vi "IDS-3060-control.vi"() -> ()   [LabVIEW 2014]
uses:
  <vilib>/Analysis/NI_AALBase.lvlib
panel:
  in  "Save image":bool
  in  "File name":string="img"
  in  "Folder Path":path=path "D:/Images/asd"
  in  "zoom":dbl(slide)=0.9914131207450079 scale=0.1..5.0
  in  "height":dbl(slide)=1272.7748691099475 scale=0.0..1300.0
  in  "width":dbl(slide)=2000.0 scale=0.0..2000.0
  out "white leve":u8=255
  out "black levell":u8
  in  "Slide":cluster{u8, u8}(slide)={0, 255} scale=0.0..255.0
  out "SizeOut":T1
  in  "stop":bool
  out "error out":errorcluster
  in  "Exposure[ms]":dbl=20.0 format="%#_13g"
  out "Hist":T2(graph)
  out "image":u8[][](graph) caption="Image"
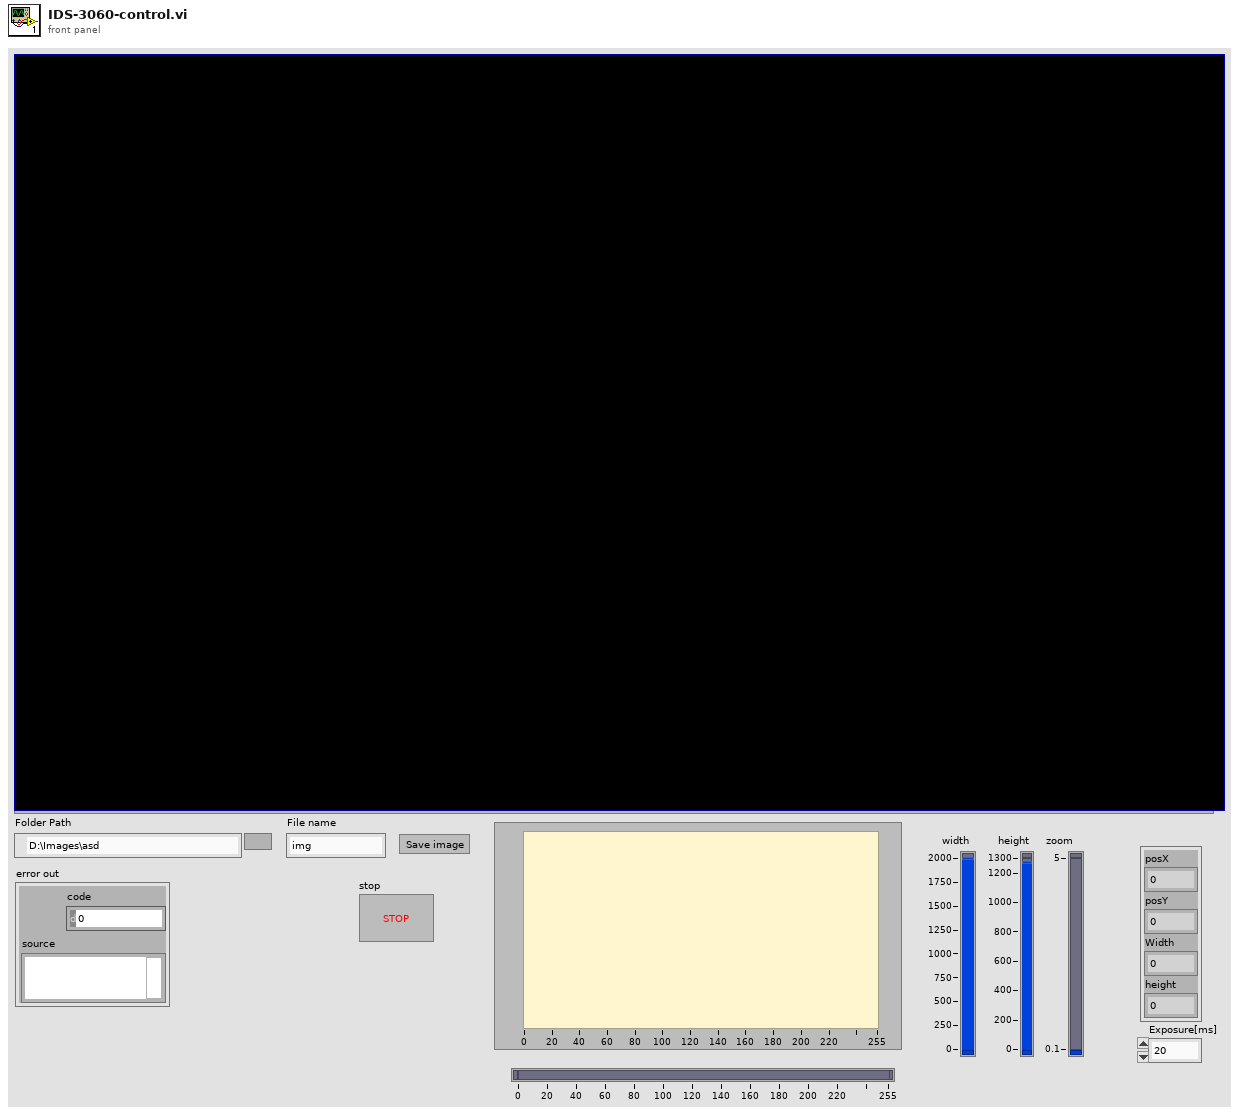
[diagram p1: front panel]
types:
  T1 = cluster{"posX":i32, "posY":i32, "Width":i32, "height":i32}
  T2 = cluster{"X Values":dbl[], "Histogram: h(x)":i32[]}
  T3 = cluster{"Rows Per Strip":i32, "Photometric":i32, "Compression Type":i32}
  T4 = typedef "IMAQ Image.ctl" = refnum<image>
  T5 = cluster{"posX":dbl, "posY":dbl, "Width":dbl, "height":dbl}
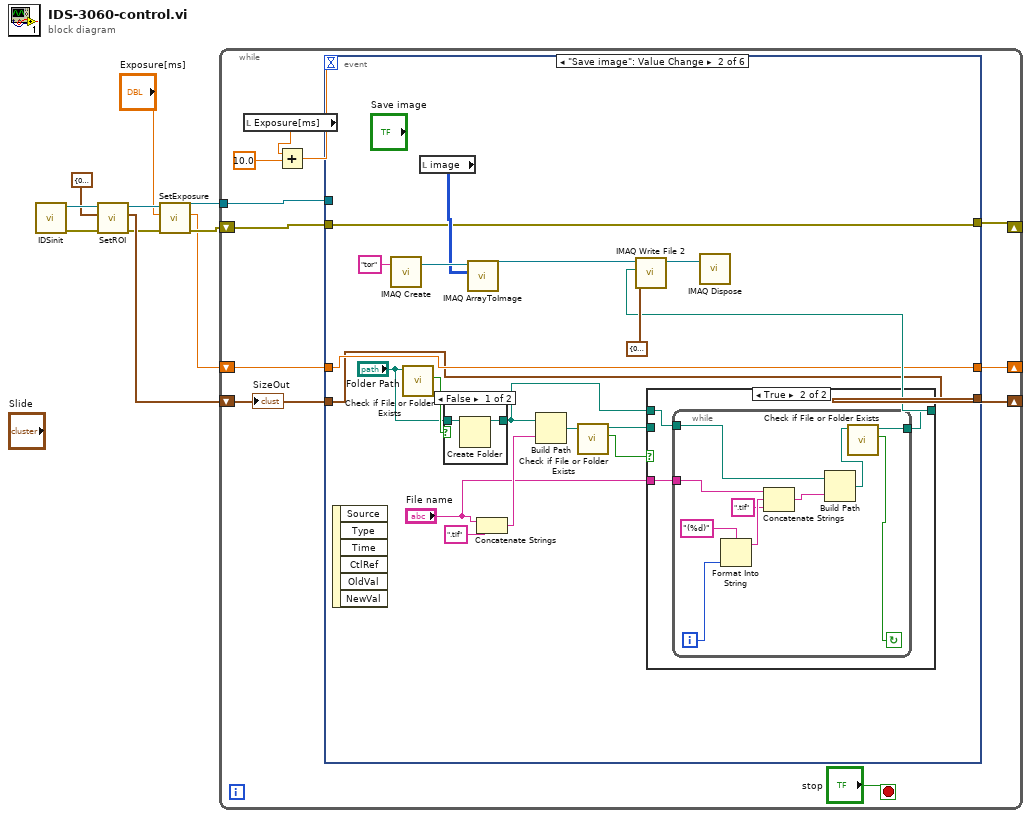
[diagram p0: block diagram]
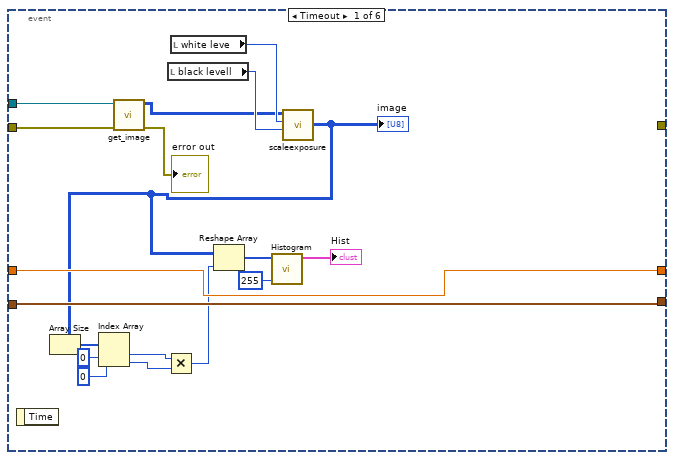
[diagram p2: hidden frame]
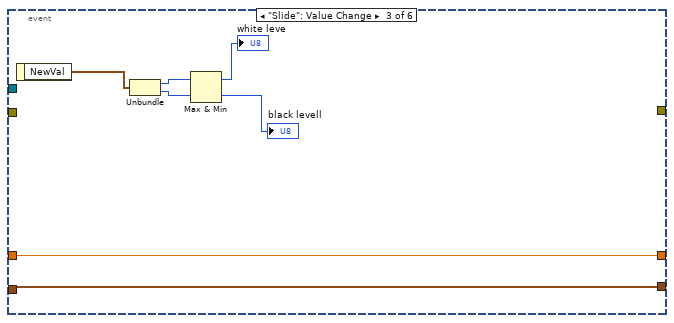
[diagram p5: hidden frame]
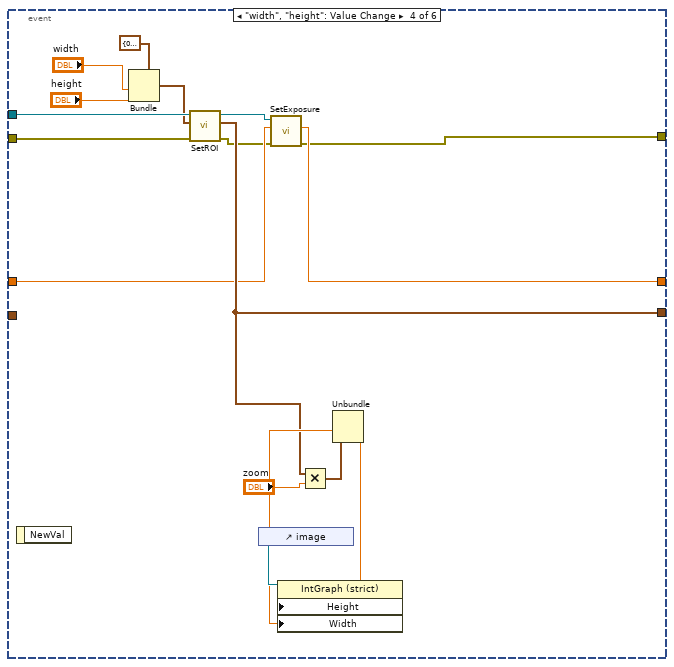
[diagram p6: hidden frame]
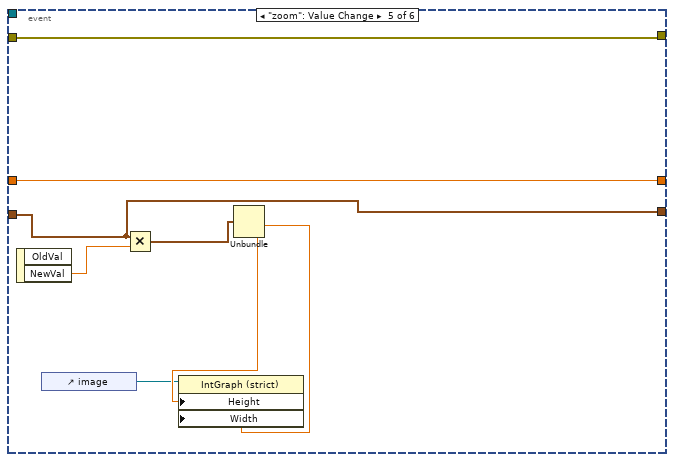
[diagram p7: hidden frame]
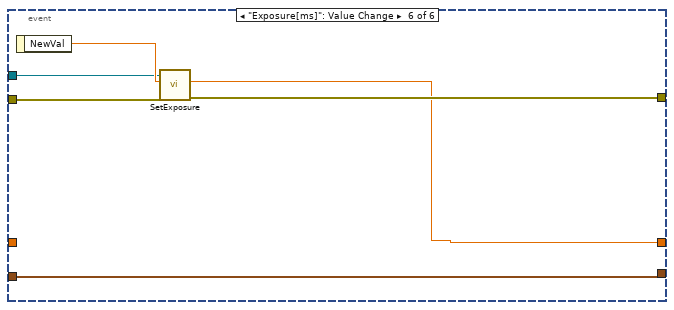
[diagram p8: hidden frame]
diagram:
  n1 = call "IDSinit.vi"() -> ("error out"=w8:errorcluster, "reference out"=w10:refnum<k24>)  [unwired: 7 in, 2 out]
  n2 = call "SetROI.vi"("error in (no error)"=w8, "SizeIn"=T1 {"posX"=0, "posY"=0, "Width"=2000, "height"=2000}, "reference in"=w10) -> ("error out"=w2:errorcluster, "SizeOut"=w5:T1, "reference out"=w9:refnum<k24>)  [unwired: 5 in]
  n3 = call "SetExposure.vi"("error in (no error)"=w2, "Exposure[ms]"="Exposure[ms]", "Reference in"=w9) -> ("error out"=w6:errorcluster, "exposure"=w1:dbl, "reference out"=w7:refnum<k24>)  [unwired: 4 in, 1 out]
  n4 = while {
    tunnel: w7 -> [w21]
    shift-right: [w19] -> _
    shift-left: w6 -> [w20]
    shift-right: [w18] -> _
    shift-left: w5 -> [w12]
    shift-right: [w13] -> _
    shift-left: w1 -> [w11]
    stop <- "stop" stop-if-true
    n5 = local read "Exposure[ms]"() -> (w16:dbl)
    n6 = Add(x=w16, y=10.0 ("Exposure[ms]")) -> (x+y=w14:dbl)
    n7 = event shown="[1] \"Save image\": Value Change" {
      selector: _ -> [_ _ _ _ _ _]
      dyn-events: _ -> [_ _ _ _ _ _]
      timeout: w14 -> [_ _ _ _ _ _]
      tunnel: w21 -> [w39 _ _ w99 _ w108]
      tunnel: w20 -> [w38 w41 _ w98 w104 w109]
      tunnel: [_ w41 _ w83 w104 w113] -> w19
      tunnel: [w33 w42 w76 w93 w100 w110] -> w18
      tunnel: w12 -> [w33 w42 w76 _ w100 w110]
      tunnel: [w32 w43 w77 w85 w106 w111] -> w13
      tunnel: w11 -> [w32 w43 w77 w86 w106 _]
      event Timeout {
        n8 = event-data() -> ()  [unwired: 1 in, 1 out]
        n9 = call "get_image.vi"("error in (no error)"=w38, "reference"=w39) -> ("error out"=→"error out":errorcluster, "Array"=w29:u8[][])  [unwired: 8 in]
        n10 = local read "black levell"() -> (w31:u8)
        n11 = local read "white leve"() -> (w30:u8)
        n12 = call "scaleexposure.vi"("black"=w31, "white"=w30, "image in"=w29) -> ("image out"=w22:u8[][])  [unwired: 8 in]
        "image" <- w22
        n13 = Array Size(array=w22) -> (size(s)=w28:i32[])
        n14 = Index Array(array=w28, index #1=0 ("index"), index #2=0 ("index")) -> (element #1=w25:i32, element #2=w24:i32)
        n15 = Multiply(x=w25, y=w24) -> (x*y=w23:i32)
        n16 = Reshape Array(w22, w23) -> (w36:u8[])
        n17 = call <vilib>:"Histogram.vi"("intervals"=255, "X"=w36) -> ("Histogram Graph"=→"Hist":T2)  [unwired: 6 in, 3 out]
      }
      event "Save image": Value Change {
        n18 = event-data() -> ()  [unwired: 1 in, 6 out]
        n19 = call "IMAQ Create"("Image Name"="tor") -> ("New Image"=w58:T4)  [unwired: 4 in, 1 out]
        n20 = call <vilib>:"Check if File or Folder Exists.vi"("path"="Folder Path") -> ("file or folder exists?"=w52:bool)  [unwired: 8 in, 2 out]
        n21 = local read "image"() -> (w56:u8[][])
        n22 = case shown="False" w52 {
          tunnel: "Folder Path" -> [w74 w75]
          tunnel: [w73 w75] -> w45
          frame False {
            n23 = Create Folder(path (use dialog)=w74) -> (created path=w73:path)  [unwired: 2 in, 2 out]
          }
          frame True {
          }
        }
        n24 = call "IMAQ ArrayToImage"("Image Pixels (U8)"=w56, "Image"=w58) -> ("Image Out"=w55:T4)  [unwired: 8 in, 1 out]
        n25 = Concatenate Strings("File name", ".tif" ("string")) -> (w49:string)
        n26 = Build Path(base path=w45, name or relative path=w49) -> (appended path=w48:path)
        n27 = call <vilib>:"Check if File or Folder Exists.vi"("path"=w48) -> ("file or folder exists?"=w40:bool, "dup path"=w47:path)  [unwired: 8 in, 1 out]
        n28 = case shown="True" w40 {
          tunnel: w47 -> [w59 _]
          tunnel: "File name" -> [_ w61]
          tunnel: [w59 w60] -> w44
          tunnel: w45 -> [_ w62]
          frame False {
          }
          frame True {
            n29 = while {
              tunnel: w62 -> [w66]
              tunnel: w61 -> [w72]
              tunnel: [w63] -> w60
              i -> [w71]
              stop <- w64 continue-if-true
              n30 = Format Into String(format string="(%d)", w71) -> (resulting string=w69:string)  [unwired: 2 in, 1 out]
              n31 = Concatenate Strings(w72, w69, ".tif" ("string")) -> (w67:string)
              n32 = Build Path(base path=w66, name or relative path=w67) -> (appended path=w65:path)
              n33 = call <vilib>:"Check if File or Folder Exists.vi"("path"=w65) -> ("file or folder exists?"=w64:bool, "dup path"=w63:path)  [unwired: 8 in, 1 out]
            }
          }
        }
        n34 = call-poly "IMAQ Write File 2"("TIFF Options"=T3 {"Rows Per Strip"=0, "Photometric"=1, "Compression Type"=0}, "File Path"=w44, "Image"=w55) -> ("Image Out (duplicate)"=w53:T4)  [unwired: 7 in, 1 out]
        n35 = call "IMAQ Dispose"("Image"=w53) -> ()  [unwired: 5 in, 1 out]
      }
      event "Slide": Value Change {
        n36 = event-data() -> ("NewVal"=w82:cluster{u8, u8})  [unwired: 1 in]
        n37 = Unbundle(w82) -> (w81:u8, w80:u8)
        n38 = Max & Min(x=w81, y=w80) -> (max(x,y)=→"white leve":u8, min(x,y)=→"black levell":u8)
      }
      event "width", "height": Value Change {
        n39 = event-data() -> ()  [unwired: 1 in, 1 out]
        n40 = Bundle(cluster=T1 {"posX"=0, "posY"=0, "Width"=0, "height"=0} ("SizeIn"), "Width"="width", "height"="height") -> (w90:T1)  [unwired: 2 in]
        n41 = call "SetROI.vi"("error in (no error)"=w98, "SizeIn"=w90, "reference in"=w99) -> ("error out"=w84:errorcluster, "SizeOut"=w93:T1, "reference out"=w87:refnum<k24>)  [unwired: 5 in]
        n42 = control-ref of="image"() -> (w97:refnum<vi>)
        n43 = call "SetExposure.vi"("error in (no error)"=w84, "Exposure[ms]"=w86, "Reference in"=w87) -> ("error out"=w83:errorcluster, "exposure"=w85:dbl)  [unwired: 4 in, 2 out]
        n44 = Multiply(x=w93, y="zoom") -> (x*y=w92:T5)
        n45 = Unbundle(w92) -> ("Width"=w95:dbl, "height"=w96:dbl)  [unwired: 2 out]
        n46 = property class="IntGraph (strict)"(reference=w97, "Height"=w96, "Width"=w95) -> ()  [unwired: 1 in, 2 out]
      }
      event "zoom": Value Change {
        n47 = event-data() -> ("NewVal"=w107:dbl)  [unwired: 1 in, 1 out]
        n48 = control-ref of="image"() -> (w101:refnum<vi>)
        n49 = Multiply(x=w100, y=w107) -> (x*y=w105:T5)
        n50 = Unbundle(w105) -> ("Width"=w102:dbl, "height"=w103:dbl)  [unwired: 2 out]
        n51 = property class="IntGraph (strict)"(reference=w101, "Height"=w103, "Width"=w102) -> ()  [unwired: 1 in, 2 out]
      }
      event "Exposure[ms]": Value Change {
        n52 = event-data() -> ("NewVal"=w112:dbl)  [unwired: 1 in]
        n53 = call "SetExposure.vi"("error in (no error)"=w109, "Exposure[ms]"=w112, "Reference in"=w108) -> ("error out"=w113:errorcluster, "exposure"=w111:dbl)  [unwired: 4 in, 2 out]
      }
    }
    "SizeOut" <- w12
  }
